vi "Measure Waveform.vi"(9 "Measured Amplitude":refnum<class "Abs_Double Float.lvclass">, 10 "Measured Frequency":refnum<class "Abs_Double Float.lvclass">, 11 "Abs_Waveform in":refnum<class "Abs_Waveform.lvclass">) -> (3 "Measure Waveform out":refnum<class "Measure Waveform.lvclass">)   [LabVIEW 2021]
uses:
  <vilib>/TSA/Abstract Data Classes/Abs_Types/Double Float/Abs_Double Float.lvclass
  Measure Waveform.lvclass
  <vilib>/TSA/Abstract Data Classes/Abs_Types/Waveform/Abs_Waveform.lvclass
  Measure Waveform.lvclass/Measure Waveform.ctl
  Properties/Write Abs_Waveform.vi
  Properties/Write Measured Frequency.vi
  Properties/Write Measured Amplitude.vi
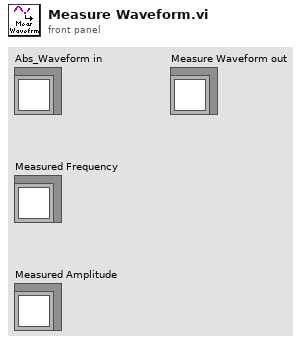
[diagram p1: front panel]
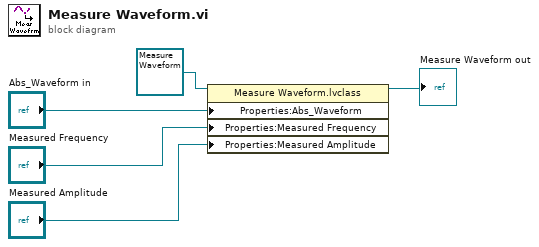
[diagram p0: block diagram]
diagram:
  n1 = property class="Measure Waveform.lvclass"(reference=refnum<class "Measure Waveform.lvclass"> refnum ("Measure Freq.lvclass"), "Properties:Abs_Waveform"="Abs_Waveform in", "Properties:Measured Frequency"="Measured Frequency", "Properties:Measured Amplitude"="Measured Amplitude") -> (reference out=→"Measure Waveform out":refnum<class "Measure Waveform.lvclass">)  [unwired: 1 in, 1 out]
